vi "SS_FPGA_Drop0.vi"() -> ()   [LabVIEW 2016]
uses:
  <vilib>/rvi/DataTransferAndStorage/Container/XNode/niFpgaContainer.xnode
  <vilib>/eio/EIONode/EIONode.xnode
  <vilib>/rvi/eio/common/nirviEmuTemplateMethod_errors.vi
  <vilib>/rvi/interface/RandomDataEmulation/nirviRandomDataFpgaReadWriteTemplate.vi
panel:
  out "error out":errorcluster
  out "Actual Duration (ms)":u32
  out "Actual Number of Samples":i32
  out "Number of Channels":i32
  in  "Scan Rate (mSec)":u32 caption="Count(mSec)"
  in  "Duration (mSec)":u32 caption="Duration (Sec)"
  out "Complete":bool
  in  "Start Acquisition":bool
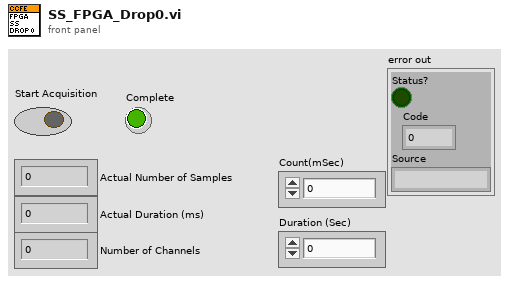
[diagram p1: front panel]
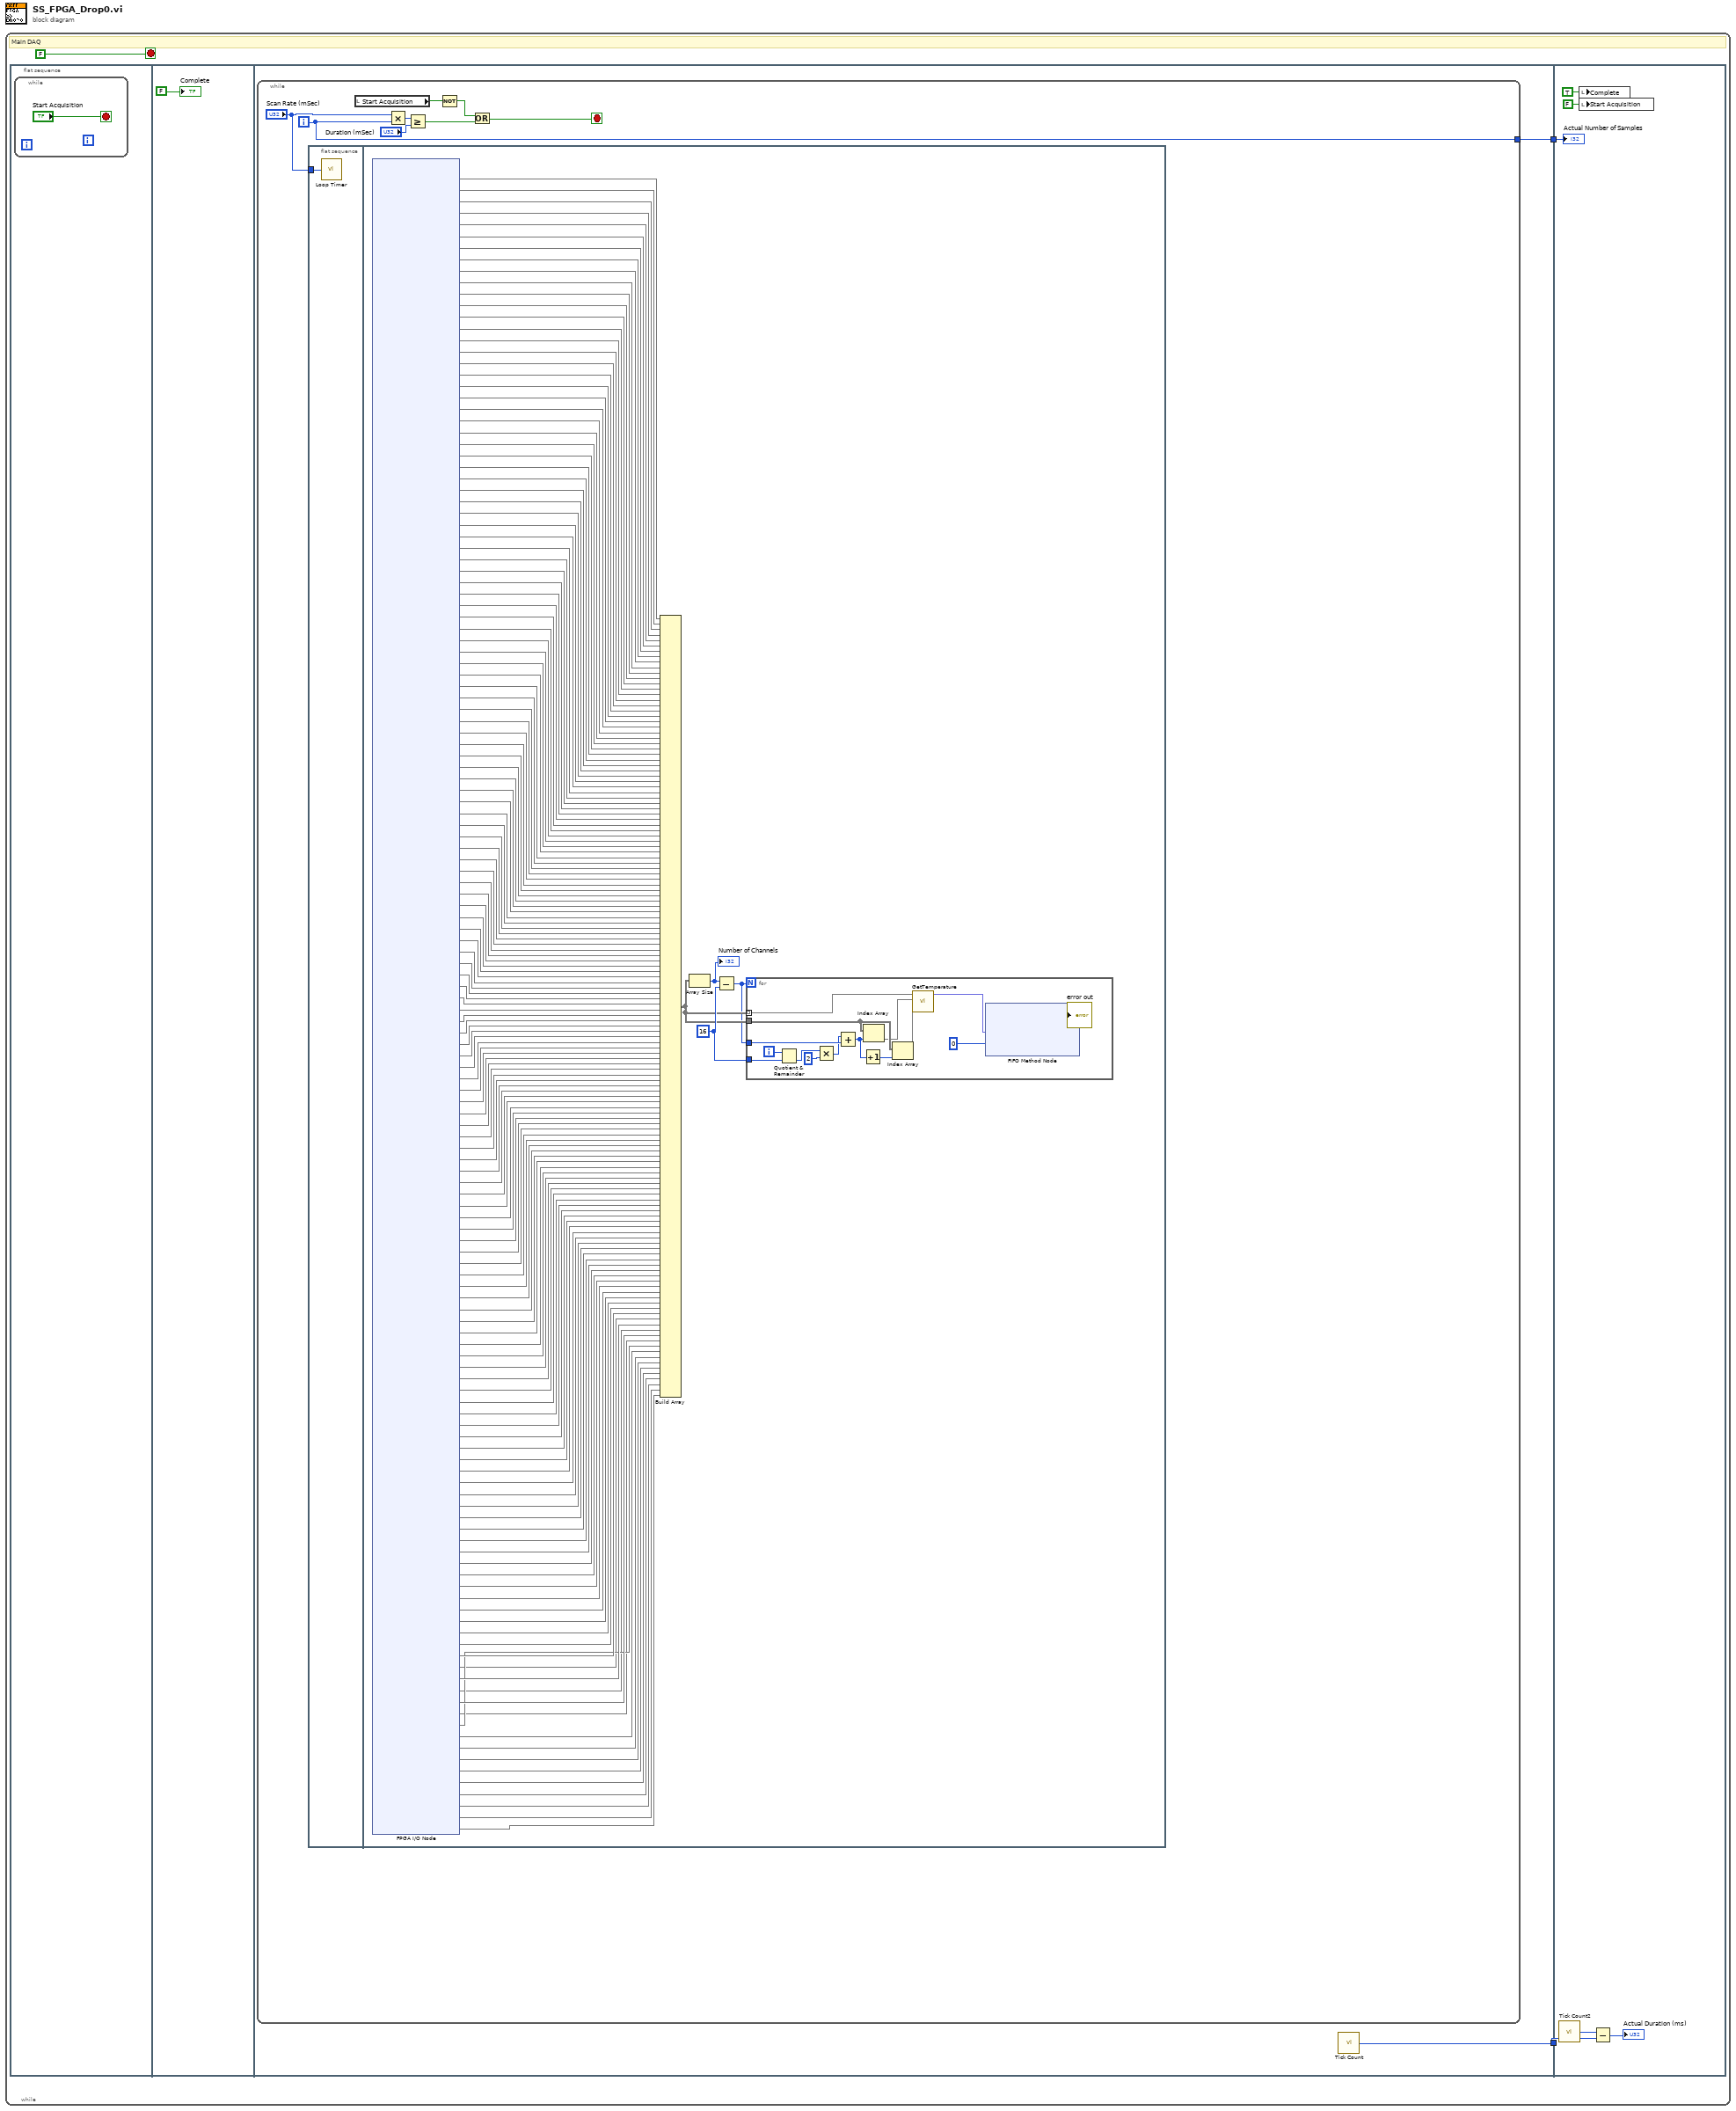
[diagram p0: block diagram]
diagram:
  n1 = while {
    stop <- FALSE ("Stop Button") stop-if-true
    # "Main DAQ"
    n2 = flat-sequence {
      tunnel: [w7] -> w2
      tunnel: [w6] -> w1
      tunnel: w2 -> [w182]
      tunnel: w1 -> [w180]
      frame #0 {
        n3 = while {
          stop <- "Start Acquisition" stop-if-true
        }
      }
      frame #1 {
        "Complete" <- FALSE
      }
      frame #2 {
        n4 = while {
          tunnel: [w9] -> w6
          i -> [w9]
          stop <- w11 stop-if-true
          n5 = flat-sequence {
            tunnel: "Scan Rate (mSec)" -> [w16]
            frame #0 {
              n6 = call "Loop Timer"("Count(mSec)"=w16) -> ()  [unwired: 1 out]
            }
            frame #1 {
              w35 = 16 ("y")
              n7 = xnode "FPGA I/O Node"() -> ("Mod1/TC0"=w164, "Mod1/TC1"=w163, "Mod1/TC2"=w162, "Mod1/TC3"=w161, "Mod1/TC4"=w160, "Mod1/TC5"=w159, "Mod1/TC6"=w158, "Mod1/TC7"=w157, "Mod1/TC8"=w156, "Mod1/TC9"=w155, "Mod1/TC10"=w154, "Mod1/TC11"=w153, "Mod1/TC12"=w152, "Mod1/TC13"=w151, "Mod1/TC14"=w150, "Mod1/TC15"=w149, "Mod2/TC0"=w148, "Mod2/TC1"=w147, "Mod2/TC2"=w146, "Mod2/TC3"=w145, "Mod2/TC4"=w144, "Mod2/TC5"=w143, "Mod2/TC6"=w142, "Mod2/TC7"=w141, "Mod2/TC8"=w140, "Mod2/TC9"=w139, "Mod2/TC10"=w138, "Mod2/TC11"=w137, "Mod2/TC12"=w136, "Mod2/TC13"=w135, "Mod2/TC14"=w134, "Mod2/TC15"=w133, "Mod3/TC0"=w132, "Mod3/TC1"=w131, "Mod3/TC2"=w130, "Mod3/TC3"=w129, "Mod3/TC4"=w128, "Mod3/TC5"=w127, "Mod3/TC6"=w126, "Mod3/TC7"=w125, "Mod3/TC8"=w124, "Mod3/TC9"=w123, "Mod3/TC10"=w122, "Mod3/TC11"=w121, "Mod3/TC12"=w120, "Mod3/TC13"=w119, "Mod3/TC14"=w118, "Mod3/TC15"=w117, "Mod4/TC0"=w116, "Mod4/TC1"=w115, "Mod4/TC2"=w114, "Mod4/TC3"=w113, "Mod4/TC4"=w112, "Mod4/TC5"=w111, "Mod4/TC6"=w110, "Mod4/TC7"=w109, "Mod4/TC8"=w108, "Mod4/TC9"=w107, "Mod4/TC10"=w106, "Mod4/TC11"=w105, "Mod4/TC12"=w104, "Mod4/TC13"=w103, "Mod4/TC14"=w102, "Mod4/TC15"=w101, "Mod5/TC0"=w100, "Mod5/TC1"=w99, "Mod5/TC2"=w98, "Mod5/TC3"=w97, "Mod5/TC4"=w96, "Mod5/TC5"=w95, "Mod5/TC6"=w94, "Mod5/TC7"=w93, "Mod5/TC8"=w92, "Mod5/TC9"=w91, "Mod5/TC10"=w90, "Mod5/TC11"=w89, "Mod5/TC12"=w88, "Mod5/TC13"=w87, "Mod5/TC14"=w86, "Mod5/TC15"=w85, "Mod6/TC0"=w84, "Mod6/TC1"=w83, "Mod6/TC2"=w82, "Mod6/TC3"=w81, "Mod6/TC4"=w80, "Mod6/TC5"=w79, "Mod6/TC6"=w78, "Mod6/TC7"=w77, "Mod6/TC8"=w76, "Mod6/TC9"=w75, "Mod6/TC10"=w74, "Mod6/TC11"=w73, "Mod6/TC12"=w72, "Mod6/TC13"=w71, "Mod6/TC14"=w70, "Mod6/TC15"=w69, "Mod7/TC0"=w68, "Mod7/TC1"=w67, "Mod7/TC2"=w66, "Mod7/TC3"=w65, "Mod7/TC4"=w64, "Mod7/TC5"=w63, "Mod7/TC6"=w62, "Mod7/TC7"=w61, "Mod7/TC8"=w60, "Mod7/TC9"=w59, "Mod7/TC10"=w58, "Mod7/TC11"=w57, "Mod7/TC12"=w56, "Mod7/TC13"=w55, "Mod7/TC14"=w54, "Mod7/TC15"=w53, "Mod8/TC0"=w52, "Mod8/TC1"=w51, "Mod8/TC2"=w50, "Mod8/TC3"=w49, "Mod8/TC4"=w48, "Mod8/TC5"=w47, "Mod8/TC6"=w46, "Mod8/TC7"=w45, "Mod8/TC8"=w44, "Mod8/TC9"=w43, "Mod8/TC10"=w42, "Mod8/TC11"=w41, "Mod8/TC12"=w40, "Mod8/TC13"=w39, "Mod8/TC14"=w38, "Mod8/TC15"=w37, "Mod1/Autozero"=w32, "Mod1/CJC"=w24, "Mod2/Autozero"=w31, "Mod2/CJC"=w23, "Mod3/Autozero"=w30, "Mod3/CJC"=w22, "Mod4/Autozero"=w29, "Mod4/CJC"=w21, "Mod5/Autozero"=w28, "Mod5/CJC"=w20, "Mod6/Autozero"=w27, "Mod6/CJC"=w19, "Mod7/Autozero"=w26, "Mod7/CJC"=w18, "Mod8/Autozero"=w25, "Mod8/CJC"=w17)  [unwired: 144 in, 144 out]
              n8 = Build Array(w164, w163, w162, w161, w160, w159, w158, w157, w156, w155, w154, w153, w152, w151, w150, w149, w148, w147, w146, w145, w144, w143, w142, w141, w140, w139, w138, w137, w136, w135, w134, w133, w132, w131, w130, w129, w128, w127, w126, w125, w124, w123, w122, w121, w120, w119, w118, w117, w116, w115, w114, w113, w112, w111, w110, w109, w108, w107, w106, w105, w104, w103, w102, w101, w100, w99, w98, w97, w96, w95, w94, w93, w92, w91, w90, w89, w88, w87, w86, w85, w84, w83, w82, w81, w80, w79, w78, w77, w76, w75, w74, w73, w72, w71, w70, w69, w68, w67, w66, w65, w64, w63, w62, w61, w60, w59, w58, w57, w56, w55, w54, w53, w52, w51, w50, w49, w48, w47, w46, w45, w44, w43, w42, w41, w40, w39, w38, w37, w32, w24, w31, w23, w30, w22, w29, w21, w28, w20, w27, w19, w26, w18, w25, w17) -> (w34:void[])
              n9 = Array Size(array=w34) -> (size(s)=w36:i32)
              "Number of Channels" <- w36
              n10 = Subtract(x=w36, y=w35) -> (x-y=w33:i32)
              n11 = for {
                N: w33 -> [_]
                tunnel: w34 -> [w177] mode=indexing
                tunnel: w35 -> [w175]
                tunnel: w34 -> [w173]
                tunnel: w33 -> [w170]
                i -> [w176]
                n12 = Quotient & Remainder(x=w176, y=w175) -> (floor(x/y)=w168:i32)  [unwired: 1 out]
                n13 = Multiply(x=w168, y=2) -> (x*y=w167:i32)
                n14 = Add(x=w167, y=w170) -> (x+y=w171:i32)
                n15 = Increment(x=w171) -> (x+1=w174:i32)
                n16 = Index Array(array=w173, index=w171) -> (element=w165)
                n17 = Index Array(array=w173, index=w174) -> (element=w166)
                n18 = call "GetTemperature.vi"("CJC"=w166, "Autozero"=w165, "Voltage"=w177) -> ("Temperature"=w178:fxp<+/-,24,12>)  [unwired: 8 in]
                n19 = xnode ("FIFO Method Node")("Element"=w178, "Timeout"=0) -> ("error out"=→"error out":errorcluster)  [unwired: 2 in, 2 out]
              }
            }
          }
          n20 = local read "Start Acquisition"() -> (w12:bool)
          n21 = Multiply(x="Scan Rate (mSec)", y=w9) -> (x*y=w15:u32)
          n22 = Greater Or Equal?(x=w15, y="Duration (mSec)") -> (x >= y?=w10:bool)
          n23 = Not(x=w12) -> (.not. x?=w13:bool)
          n24 = Or(x=w13, y=w10) -> (x .or. y?=w11:bool)
        }
        n25 = call "Tick Count"() -> ("Tick Count(mSec)"=w7:u32)
      }
      frame #3 {
        n26 = call "Tick Count2"() -> ("Tick Count(mSec)"=w183:u32)
        n27 = local write "Complete"(TRUE ("Complete")) -> ()
        n28 = local write "Start Acquisition"(FALSE ("Start Acquisition")) -> ()
        n29 = Subtract(x=w183, y=w182) -> (x-y=→"Actual Duration (ms)":u32)
        "Actual Number of Samples" <- w180
      }
    }
  }
